vi "Day 1-2.vi"() -> ()   [LabVIEW 2022 SP3]
uses:
  <vilib>/regexp/Match Regular Expression.xnode
panel:
  out "sum":i32
  out "Array":i32[](array[numeric])
  out "string array":string[](array[string])
  in  "String":string="46threevqs8114\nthreetwoonez1gtrd\n6ffxbtff\n769twotwo6rv9\ngjrcjrkvghthreegqqrg82qbct\nzkxjhgprtrlcfeight795five8\n99seven3vdcgvmvxtjtwodc5\nthree5eightthree3four3vtkkqrgxs\nfour863mrrnrsxrkone\nsevenntgvnrrqfvxh2ttnkgffour8fiveone\n49fbsfb\n3rbmlsksg\nztgszqjjsrtmgqx6572\n3bqnfxkdbonesixseven\nmfgx32ftpbhgngm7\nfzrpfhbfvj6dbxbtfs7twofksfbshrzkdeightwoqg\n2xcftwo\ncshmmltsml4fiveeightdn\neightthsix1\ntwo1gvfxcqnrfnbeightthreexznhbmmk\n3917sevenvxqxntcgxskh\nksctcnfxdsk96drlbjkthreesfqlvnpvfbcbmg\n8nvrmzfs46\n5dbgltmgg1xvtqfkdxsrxzltwo1pgqlqndlc\neight7four6rpbtmjzj5\n41seven\ngpmfhninexxgqr6\n15sixdrhxzcmqf\n8fivettgmcs..."
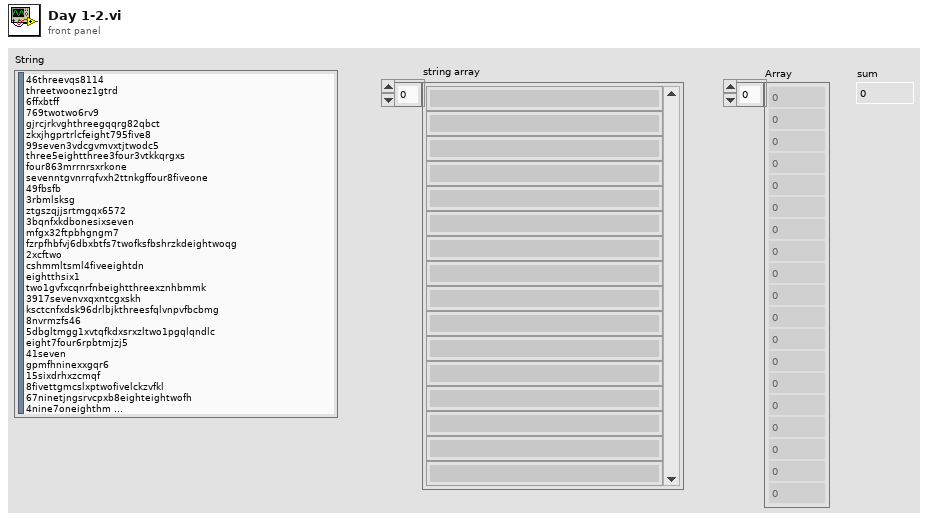
[diagram p1: front panel]
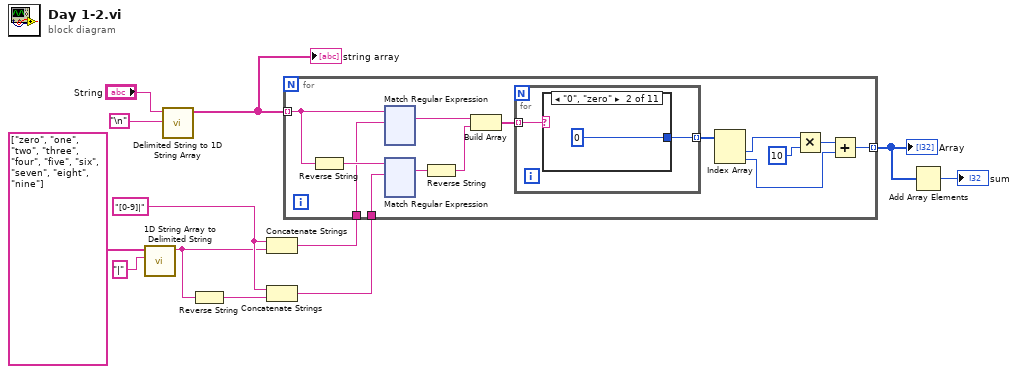
[diagram p0: block diagram]
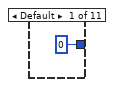
[diagram p2: hidden frame]
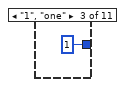
[diagram p3: hidden frame]
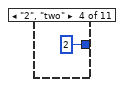
[diagram p4: hidden frame]
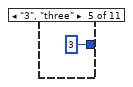
[diagram p5: hidden frame]
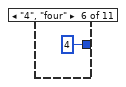
[diagram p6: hidden frame]
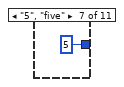
[diagram p7: hidden frame]
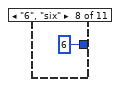
[diagram p8: hidden frame]
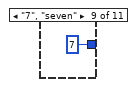
[diagram p9: hidden frame]
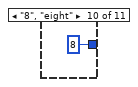
[diagram p10: hidden frame]
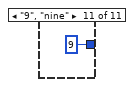
[diagram p11: hidden frame]
diagram:
  w4 = "[0-9]|"
  n1 = call <vilib>:"1D String Array to Delimited String.vi"("delimiter"="|", "string array"=string[] ["zero", "one", "two", "three", "four", "five", "six", "seven", "eight", "nine"]) -> ("delimited string"=w3:string)  [unwired: 9 in]
  n2 = call <vilib>:"Delimited String to 1D String Array.vi"("delimiter"="\n", "delimited string"="String") -> ("string array"=w10:string[])  [unwired: 9 in]
  "string array" <- w10
  n3 = Reverse String(1:w3) -> (0:w6:string)
  n4 = Concatenate Strings(w4, w3) -> (w2:string)
  n5 = Concatenate Strings(w4, w6) -> (w1:string)
  n6 = for {
    tunnel: w10 -> [w23] mode=indexing
    tunnel: [w24] -> w9 mode=indexing
    tunnel: w2 -> [w21]
    tunnel: w1 -> [w20]
    n7 = Reverse String(1:w23) -> (0:w22:string)
    n8 = xnode "Match Regular Expression"("input string"=w23, "regular expression"=w21) -> ("whole match"=w18:string)  [unwired: 4 in, 4 out]
    n9 = xnode "Match Regular Expression"("input string"=w22, "regular expression"=w20) -> ("whole match"=w19:string)  [unwired: 4 in, 4 out]
    n10 = Reverse String(1:w19) -> (0:w17:string)
    n11 = Build Array(w18, w17) -> (w16:string[])
    n12 = for {
      tunnel: w16 -> [w28] mode=indexing
      tunnel: [w27] -> w15 mode=indexing
      n13 = case shown="\"0\", \"zero\"" w28 {
        tunnel: [0 0 1 2 3 4 5 6 7 8 9] -> w27
        frame Default {
        }
        frame "0", "zero" {
        }
        frame "1", "one" {
        }
        frame "2", "two" {
        }
        frame "3", "three" {
        }
        frame "4", "four" {
        }
        frame "5", "five" {
        }
        frame "6", "six" {
        }
        frame "7", "seven" {
        }
        frame "8", "eight" {
        }
        frame "9", "nine" {
        }
      }
    }
    n14 = Index Array(array=w15) -> (element #1=w14:i32, element #2=w13:i32)  [unwired: 2 in]
    n15 = Multiply(x=w14, y=10) -> (x*y=w25:i32)
    n16 = Add(x=w25, y=w13) -> (x+y=w24:i32)
  }
  "Array" <- w9
  n17 = Add Array Elements(numeric array=w9) -> (sum=→"sum":i32)
